vi "Initialize Hardware Maestro.vi"(8 "error in (no error)":errorcluster, 10 "Hardware Maestro Config":T1) -> (0 "error out":errorcluster, 1 "Maestro Online":bool, 2 "Hardware Maestro Config 2":T1, 3 "connection ID":refnum<k5>)   [LabVIEW 2021, in "Maestro Acq.lvclass"]
doc: "Initialize the hardware references."
uses:
  Maestro Acq.lvclass
  Hardware Maestro Config.ctl
  5c305276-9a05-49e5-860c-17deb3e20d14.vi
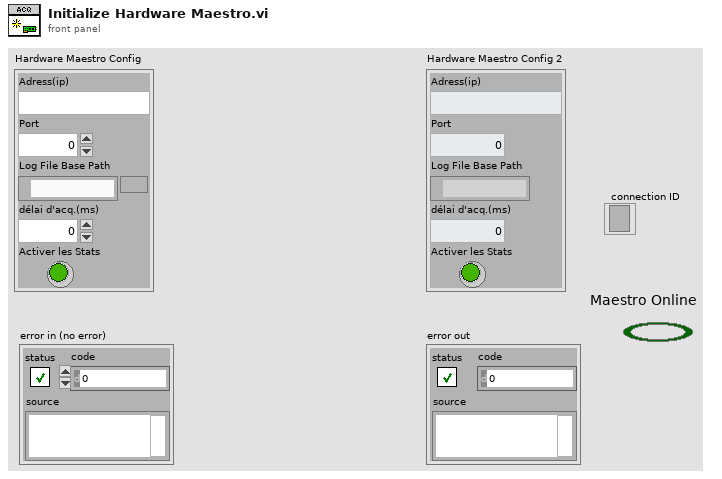
[diagram p1: front panel]
types:
  T1 = typedef "Maestro Acq.lvclass/Hardware Maestro Config.ctl" = cluster{"Adress(ip)":string, "Port":i16, "Log File Base Path":path, "délai d'acq.(ms)":i32, "Activer les Stats":bool}
  T2 = enum16{"Standard", "Buffered", "CRLF", "Immediate"}
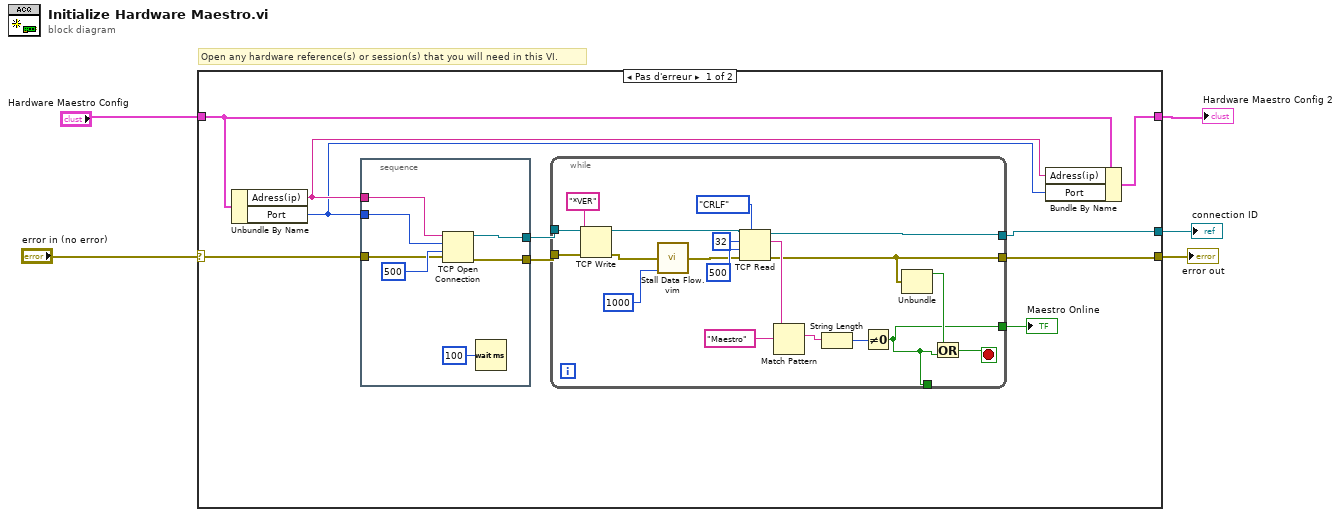
[diagram p0: block diagram]
diagram:
  # "Open any hardware reference(s) or session(s) that you will need in this VI."
  n1 = case shown="Pas d'erreur" "error in (no error)" {
    selector: "error in (no error)" -> [w10 w43]
    tunnel: [w11 w43] -> w4
    tunnel: [w15 w42] -> w2
    tunnel: "Hardware Maestro Config" -> [w14 w42]
    tunnel: [w7 _] -> w1
    frame No Error {
      n2 = Unbundle By Name(w14) -> ("Adress(ip)"=w9:string, "Port"=w8:i16)
      n3 = stacked-sequence {
        tunnel: [w41] -> w13
        tunnel: [w40] -> w12
        tunnel: w9 -> [w37]
        tunnel: w8 -> [w36]
        tunnel: w10 -> [w35]
        frame #0 {
          n4 = TCP Open Connection(address=w37, remote port or service name=w36, timeout ms (60000)=500, error in (no error)=w35) -> (connection ID=w41:refnum<k5>, error out=w40:errorcluster)  [unwired: 1 in]
          n5 = Wait (ms)(milliseconds to wait=u32 100) -> ()  [unwired: 1 out]
        }
      }
      n6 = while {
        tunnel: [w34] -> w7
        tunnel: [w21] -> w11
        tunnel: w13 -> [w33]
        tunnel: w12 -> [w32]
        tunnel: [w19] -> _
        tunnel: [w19] -> w6
        stop <- w20 stop-if-true
        n7 = TCP Write(connection ID=w33, data in="*VER" ("string"), error in (no error)=w32) -> (connection ID out=w23:refnum<k5>, error out=w18:errorcluster)  [unwired: 1 in, 1 out]
        n8 = call "Stall Data Flow.vim"("value in"=w18, "milliseconds to wait"=u32 1000) -> ("value out"=w17:errorcluster)  [unwired: 1 out]
        n9 = TCP Read(connection ID=w23, bytes to read=32, error in (no error)=w17, 7:T2."CRLF" ("mode (standard)"), 9:500 ("timeout ms (25000)")) -> (connection ID out=w34:refnum<k5>, data out=w28:string, error out=w21:errorcluster)
        n10 = Match Pattern(string=w28, regular expression="Maestro") -> (match substring=w25:string)  [unwired: 1 in, 3 out]
        n11 = String Length(string=w25) -> (length=w26:i32)
        n12 = Not Equal To 0?(x=w26) -> (x != 0?=w19:bool)
        n13 = Unbundle(w21) -> ("status"=w22:bool)  [unwired: 2 out]
        n14 = Or(x=w22, y=w19) -> (x .or. y?=w20:bool)
      }
      "Maestro Online" <- w6
      n15 = Bundle By Name(cluster=w14, "Adress(ip)"=w9, "Port"=w8) -> (w15:T1)
    }
    frame Error {
    }
  }
  "error out" <- w4
  "Hardware Maestro Config 2" <- w2
  "connection ID" <- w1
